vi "Constants.vi"() -> ()   [LabVIEW 2019, in "OPC UA Client Addon Shared.lvlib"]
doc: "Use this Global VI to access the GUIDs assigned to the page resources of the Custom Device."
uses:
  OPC UA Client Addon Shared.lvlib
panel:
  in  "Tab Control":enum32{"GUIDS", "Constants", "Properties"}(tab)=enum."Constants"
  in  "Data Array_Read.GUID":string="6479b41d-0e3c-49b5-aedf-866cd23fb01f"
  in  "Data Array_Write.GUID":string="f3b36dbc-3261-4b65-ab5a-798453c3ee28"
  in  "Data Array Tag_Read.GUID":string="08a883f4-5c65-48b3-a5df-4895967c7758"
  in  "Data Array Tag_Write.GUID":string="3e79f943-56fb-48fe-83a8-f205399ffca9"
  in  "Status Channel.GUID":string="a46ed73d-ea23-4412-b593-60d5aae521a2"
  in  "Poll Lists.GUID":string="5798e698-3e20-4276-a35f-d8622b341929"
  in  "Poll List.GUID":string="7d8844d8-8471-4553-8891-822d4ff301ba"
  in  "Offline Data Folder.GUID":string="d68d3a8e-e073-4529-90c0-4eca5eb477b1"
  in  "OPC UA Client Disable.GUID":string="f6414441-41fc-4e4d-ba9d-63aca55f0f7b"
  in  "Data Tag_Write.GUID":string="ddff34a8-6f1a-4889-ab9a-0bec442b9af9"
  in  "Data Folder.GUID":string="6579feb5-1219-4a78-b605-46d71edd99ff"
  in  "Data Tag_Read.GUID":string="d90b1919-b5dd-4572-8e65-61ab77e1880c"
  in  "Tags.GUID":string="8ca7cb8f-b8e0-4777-98b2-189d42350187"
  in  "Status.GUID":string="7edfa8db-1108-4455-b477-d5a5949050b3"
  in  "OPC UA Client.GUID":string="b427fdee-6f3d-4280-85b2-59e4741516b9"
  out "Error Codes":cluster{"number":i32, "trimmed string":string}[](array[cluster])=[{"number"=0, "trimmed string"="<0> No Error."}, {"number"=-356739, "trimmed string"="<-356739> An OPC UA server is already created."}, {"number"=-356738, "trimmed string"="<-356738> The data type or node type of the normal state node is invalid."}, {"number"=-356737, "trimmed string"="<-356737> The data type or node type of the input node is invalid."}, {"number"=-356736, "trimmed string"="<-356736> The data type or node type of the setpoint node is invalid."}, {"number"=-356735, "trimmed string"="<-356735> The data type or node type of the source node is invalid."}, {"number"=-356734, "trimmed string"="<-356734> The node ID of the notifier does not exist."}, {"number"=-356733, "trimmed string"="<-356733> The node name is invalid."}, {"number"=-356732, "trimmed string"="<-356732> The data type of the input node does not match the data type of the normal state node."}, {"number"=-356731, "trimmed string"="<-356731> The ID of the input node is invalid."}, {"number"=-356730, "trimmed string"="<-356730> The ID of the normal state node is invalid."}, {"number"=-356729, "trimmed string"="<-356729> The ID of the setpoint node is invalid."}, {"number"=-356727, "trimmed string"="<-356727> The license is not activated."}, {"number"=-356726, "trimmed string"="<-356726> The limit values do not follow: highhighLimit > highLimit > lowLimit > lowlowLimit."}, {"number"=-356725, "trimmed string"="<-356725> The historical data queue size must be larger than 0."}, {"number"=-356724, "trimmed string"="<-356724> The condition type is not supported."}, {"number"=-356723, "trimmed string"="<-356723> The condition type is unknown."}, {"number"=-356722, "trimmed string"="<-356722> The event ID is invalid."}, {"number"=-356721, "trimmed string"="<-356721> The parent node is not a notifier node."}, {"number"=-356720, "trimmed string"="<-356720> The parent node is not a folder node."}, {"number"=-356719, "trimmed string"="<-356719> The unregister refnum failed."}, {"number"=-356718, "trimmed string"="<-356718> The register refnum failed."}, {"number"=-356717, "trimmed string"="<-356717> The property value cannot be written after the OPC UA server starts."}, {"number"=-356716, "trimmed string"="<-356716> Internal error. The property node ID is invalid."}, {"number"=-356715, "trimmed string"="<-356715> Internal error. The condition node refnum is invalid."}, {"number"=-356714, "trimmed string"="<-356714> The subscription ID refers to other types of subscription."}, {"number"=-356706, "trimmed string"="<-356706> Failed to copy the certificate file to the certificate store because access is denied."}, {"number"=-356705, "trimmed string"="<-356705> Failed to create certificate store because access is denied."}, {"number"=-356704, "trimmed string"="<-356704> Failed to create certificate files because access is denied."}, {"number"=-356702, "trimmed string"="<-356702> The OPC UA server has reached the maximum number of subscriptions allowed."}, {"number"=-356701, "trimmed string"="<-356701> The port you specified for creating the server is occupied."}, {"number"=-356700, "trimmed string"="<-356700> The OPC UA server is not running."}, {"number"=-356699, "trimmed string"="<-356699> LabVIEW cannot find the certificate or private key file."}, {"number"=-356698, "trimmed string"="<-356698> Unable to locate the host."}, {"number"=-356697, "trimmed string"="<-356697> The OPC UA client failed to establish a secure connection to the OPC UA server."}, {"number"=-356696, "trimmed string"="<-356696> Value in the OPC UA server contains a syntax error."}, {"number"=-356695, "trimmed string"="<-356695> The OPC UA server does not support the specified security policy."}, {"number"=-356694, "trimmed string"="<-356694> The OPC UA server does not support the specified message mode."}, {"number"=-356688, "trimmed string"="<-356688> The ID of the source node is invalid."}, {"number"=-356683, "trimmed string"="<-356683> The requested operation is not supported or one or more parameter specified in the requested operation are not supported."}, {"number"=-356677, "trimmed string"="<-356677> The node path refers to a node that does not exist in the server address space."}, {"number"=-356676, "trimmed string"="<-356676> The OPC UA server cannot recognize the node in the request of the OPC UA client."}, {"number"=-356653, "trimmed string"="<-356653> The status of the OPC UA server is uncertain."}, {"number"=-356650, "trimmed string"="<-356650> The view version is not available or is not supported."}, {"number"=-356648, "trimmed string"="<-356648> The view timestamp is not available or is not supported."}, {"number"=-356647, "trimmed string"="<-356647> The view ID does not refer to a valid view node."}, {"number"=-356646, "trimmed string"="<-356646> The user does not have permission to perform the requested operation."}, {"number"=-356645, "trimmed string"="<-356645> The OPC UA client cannot recognize the response from the OPC UA server."}, {"number"=-356644, "trimmed string"="<-356644> An unexpected error occurred."}, {"number"=-356643, "trimmed string"="<-356643> The request cannot be processed because the request specified too many operations."}, {"number"=-356642, "trimmed string"="<-356642> Invalid timestamp in the OPC UA client request."}, {"number"=-356641, "trimmed string"="<-356641> The operation timed out."}, {"number"=-356640, "trimmed string"="<-356640> The subscription ID is not valid."}, {"number"=-356639, "trimmed string"="<-356639> The operation was cancelled because the application is shutting down."}, {"number"=-356638, "trimmed string"="<-356638> The session cannot be used because you have not activated this session."}, {"number"=-356637, "trimmed string"="<-356637> The session has been closed by the OPC UA client."}, {"number"=-356636, "trimmed string"="<-356636> The OPC UA client failed to close a session."}, {"number"=-356635, "trimmed string"="<-356635> The OPC UA server does not support the requested service."}, {"number"=-356634, "trimmed string"="<-356634> The server URI is not valid."}, {"number"=-356633, "trimmed string"="<-356633> You cannot complete the operation before you connect the OPC UA client to the OPC UA server."}, {"number"=-356632, "trimmed string"="<-356632> The OPC UA server has stopped and cannot process any requests."}, {"number"=-356631, "trimmed string"="<-356631> An error occurred when the OPC UA server was verifying the security message of the OPC UA client."}, {"number"=-356630, "trimmed string"="<-356630> The secure channel you specified is no longer valid."}, {"number"=-356629, "trimmed string"="<-356629> An operating system resource is not available."}, {"number"=-356628, "trimmed string"="<-356628> The header for the request is missing or invalid."}, {"number"=-356627, "trimmed string"="<-356627> The OPC UA client cannot read the response message from the OPC UA server, because the message size exceeds the specified limits."}, {"number"=-356626, "trimmed string"="<-356626> The OPC UA server cannot read the request message from the OPC UA client, because the message size exceeds the specified limits."}, {"number"=-356625, "trimmed string"="<-356625> The OPC UA client has cancelled the request."}, {"number"=-356624, "trimmed string"="<-356624> Not enough memory to complete this operation."}, {"number"=-356623, "trimmed string"="<-356623> No operation executed because the OPC UA client passed a list of operations with no elements."}, {"number"=-356622, "trimmed string"="<-356622> The nonce does not appear to be a random value or is not correct in length."}, {"number"=-356621, "trimmed string"="<-356621> The timestamp is out of the range the OPC UA server allows."}, {"number"=-356620, "trimmed string"="<-356620> The operation cannot complete."}, {"number"=-356619, "trimmed string"="<-356619> The OPC UA server failed to validate one or more parameters in the OPC UA client request."}, {"number"=-356618, "trimmed string"="<-356618> The OPC UA client cannot connect to the OPC UA server because the OPC UA server rejected the security policy, username, or password."}, {"number"=-356617, "trimmed string"="<-356617> The OPC UA client cannot connect to the OPC UA server because the security policy, username, or password is invalid."}, {"number"=-356616, "trimmed string"="<-356616> The message encoding and decoding limits imposed by the stack have been exceeded."}, {"number"=-356615, "trimmed string"="<-356615> Encoding halted because of invalid data in the serialized objects."}, {"number"=-356614, "trimmed string"="<-356614> Decoding halted because of invalid data in the stream."}, {"number"=-356613, "trimmed string"="<-356613> The extension object cannot be serialized or deserialized because the data type ID is not recognized."}, {"number"=-356612, "trimmed string"="<-356612> A communication problem occurred."}, {"number"=-356611, "trimmed string"="<-356611> You cannot use the certificate for the requested operation."}, {"number"=-356610, "trimmed string"="<-356610> The receiver does not trust the certificate of the sender."}, {"number"=-356609, "trimmed string"="<-356609> The certificate URI in the OPC UA client request does not match the certificate URI that the OPC UA server expects."}, {"number"=-356608, "trimmed string"="<-356608> The certificate has expired or is not yet valid."}, {"number"=-356607, "trimmed string"="<-356607> The certificate has been revoked."}, {"number"=-356606, "trimmed string"="<-356606> Unable to determine if the certificate has been revoked."}, {"number"=-356605, "trimmed string"="<-356605> The certificate provided by the OPC UA client is not valid."}, {"number"=-356603, "trimmed string"="<-356603> An issuer certificate has expired or is not yet valid."}, {"number"=-356602, "trimmed string"="<-356602> You cannot use the issuer certificate for the requested operation."}, {"number"=-356601, "trimmed string"="<-356601> Unable to determine if the issuer certificate has been revoked."}, {"number"=-356600, "trimmed string"="<-356600> The host name that you use to connect to an OPC UA server does not match a host name in the certificate."}, {"number"=-356530, "trimmed string"="<-356530> The syntax of node path is incorrect."}, {"number"=-356529, "trimmed string"="<-356529> You must select at least one security policy."}, {"number"=-356528, "trimmed string"="<-356528> You cannot remove a certificate when the OPC UA server is running."}, {"number"=-356527, "trimmed string"="<-356527> You cannot add a certificate when the OPC UA server is running."}, {"number"=-356526, "trimmed string"="<-356526> The initial value of a node in the OPC UA server address space is uncertain."}, {"number"=-356525, "trimmed string"="<-356525> The sensor from which the value is derived by the device or data source failed."}, {"number"=-356524, "trimmed string"="<-356524> The device or data source that generates the value failed."}, {"number"=-356523, "trimmed string"="<-356523> The node you want to delete does not exist in the address space."}, {"number"=-356522, "trimmed string"="<-356522> You cannot add a node when the OPC UA server is running."}, {"number"=-356521, "trimmed string"="<-356521> You cannot delete a node when the OPC UA server is running."}, {"number"=-356520, "trimmed string"="<-356520> Unable to remove one or more certificate files."}, {"number"=-356519, "trimmed string"="<-356519> Unable to add one or more certificate files."}, {"number"=-356517, "trimmed string"="<-356517> OPC UA client refnum in is not valid."}, {"number"=-356516, "trimmed string"="<-356516> OPC UA server refnum in is not valid."}, {"number"=-356515, "trimmed string"="<-356515> The data type of the node does not match the data type of the value to write."}, {"number"=-356514, "trimmed string"="<-356514> The data type of the node does not match the expected data type."}, {"number"=-356512, "trimmed string"="<-356512> An error occurred when writing to the node."}, {"number"=-356511, "trimmed string"="<-356511> An error occurred when reading the node."}, {"number"=-356510, "trimmed string"="<-356510> The OPC UA server does not support this feature."}, {"number"=-356509, "trimmed string"="<-356509> The node you want to add already exists in the address space."}, {"number"=-356508, "trimmed string"="<-356508> Unable to add a node to the address space."}, {"number"=-356507, "trimmed string"="<-356507> Unable to add a property to the address space."}, {"number"=-356506, "trimmed string"="<-356506> Unable to add an item to the address space."}, {"number"=-356505, "trimmed string"="<-356505> Unable to add a folder to the address space."}, {"number"=-356504, "trimmed string"="<-356504> Unable to find a node in the address space."}, {"number"=-356503, "trimmed string"="<-356503> This node does not support read and write operations."}, {"number"=-356502, "trimmed string"="<-356502> Not enough memory to complete this operation."}, {"number"=-356500, "trimmed string"="<-356500> An internal error occurred as a result of a programming or configuration error."}, {"number"=356501, "trimmed string"="<356501> Because historical access is not enabled, setting the queue size does not activate historical access."}, {"number"=356502, "trimmed string"="<356502> The severity level range is from 1 to 1000."}, {"number"=356503, "trimmed string"="<356503> The high high severity level should be greater than the high severity level while the low low severity level should be less than the low severity level."}]
  in  "Refs.Status":string="Statuses"
  in  "Status.ErrorCode":string="Poll Engine Error Code"
  in  "Status.BadTags":string="Bad Tags"
  in  "Status.GoodTags":string="Good Tags"
  in  "Status.TotalTags":string="Total Tags"
  in  "Poll Lists.Name":string="Poll Lists"
  in  "Poll List.Name":string="Poll List"
  in  "Offline Data Folder.Name":string="Channel Folder"
  in  "Tags.Name":string="Tags"
  in  "Status.Name":string="Status"
  in  "Channel.Access":string="DataAccess"
  in  "Compiled.Settings":string="Compiled Settings"
  in  "Poll.Rate":string="PollRate"
  in  "Connect.IP":string="IP"
  in  "Connect.Port":string="Connect.Port"
  in  "Connect.User":string="User"
  in  "Connect.Password":string="Password"
  in  "Connect.MessageMode":string="MessageMode"
  in  "Connect.Security":string="Security"
  in  "Connect.ClientCert.Public":string="ClientPublicCert"
  in  "Connect.ServerCert":string="ServerCert"
  in  "Connect.ClientCert.Private":string="ClientPrivateCert"
  in  "Channel.DataType":string="DataType"
  in  "Channel.TagPath":string="TagPath"
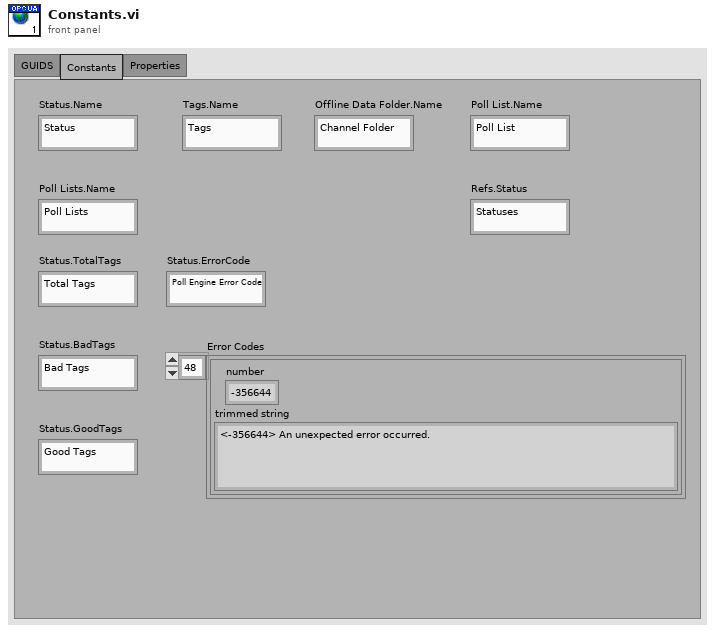
[diagram p1: front panel]
diagram:
